vi "UniqueNameDialog.vi"(9 "Names in use":string[](array[string]), 10 "Device Name":string) -> (2 "Unique name":string)   [LabVIEW 2013]
doc: "Present dialog to ask for unique name, showing user list of reserved names."
uses:
  <vilib>/Utility/miscctls.llb/LVSelectionTypeDef.ctl
panel:
  out "unique?":bool
  in  "OK button":bool
  # "Please enter a unique name:"
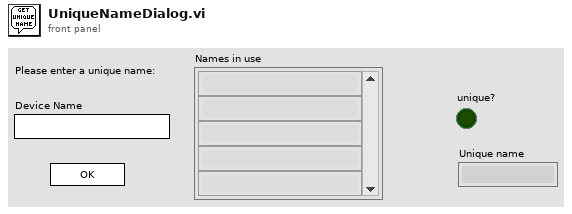
[diagram p1: front panel]
types:
  T1 = typedef "LVSelectionTypeDef.ctl" = cluster{"Selection Start":u32, "Selection End":u32}
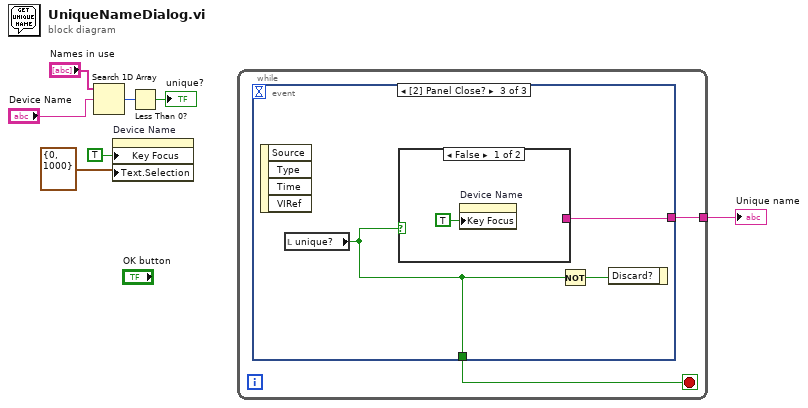
[diagram p0: block diagram]
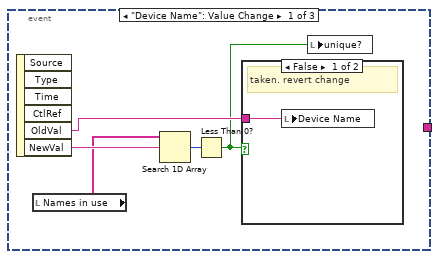
[diagram p2: hidden frame]
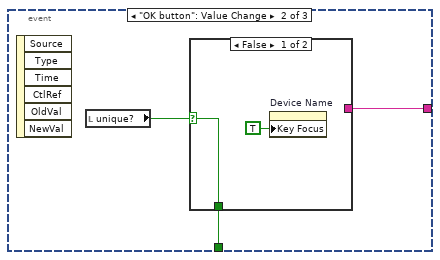
[diagram p4: hidden frame]
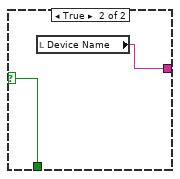
[diagram p5: hidden frame]
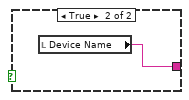
[diagram p6: hidden frame]
diagram:
  n1 = Search 1D Array(1D array="Names in use", element="Device Name") -> (index of element=w4:i32)  [unwired: 1 in]
  n2 = property on="Device Name" class="Str"("Key Focus"=TRUE, "Text.Selection"=T1 {"Selection Start"=0, "Selection End"=1000}) -> ()  [unwired: 2 in, 2 out]
  n3 = Less Than 0?(x=w4) -> (x < 0?=→"unique?":bool)
  n4 = while {
    tunnel: [w8] -> w7
    stop <- w9 stop-if-true
    n5 = event shown="[2] Panel Close?" {
      selector: _ -> [_ _ _]
      dyn-events: _ -> [_ _ _]
      timeout: _ -> [_ _ _]
      tunnel: [_ w16 w23] -> w9
      tunnel: [_ w17 w25] -> w8
      event "Device Name": Value Change {
        n6 = event-data() -> ("OldVal"=w11:string, "NewVal"=w14:string)  [unwired: 1 in, 4 out]
        n7 = local read "Names in use"() -> (w13:string[])
        n8 = Search 1D Array(1D array=w13, element=w14) -> (index of element=w12:i32)  [unwired: 1 in]
        n9 = Less Than 0?(x=w12) -> (x < 0?=w10:bool)
        n10 = case shown="False" w10 {
          tunnel: w11 -> [w15 _]
          frame False {
            # "taken. revert change"
            n11 = local write "Device Name"(w15) -> ()
          }
          frame True {
            # "unique!"
          }
        }
        n12 = local write "unique?"(w10) -> ()
      }
      event "OK button": Value Change {
        n13 = event-data() -> ()  [unwired: 1 in, 6 out]
        n14 = local read "unique?"() -> (w18:bool)
        n15 = case shown="False" w18 {
          selector: w18 -> [w19 w22]
          tunnel: [_ w21] -> w17
          tunnel: [w19 w22] -> w16
          frame False {
            n16 = property on="Device Name" class="Str"("Key Focus"=TRUE) -> ()  [unwired: 2 in, 2 out]
          }
          frame True {
            n17 = local read "Device Name"() -> (w21:string)
          }
        }
      }
      event Panel Close? {
        n18 = event-data() -> ()  [unwired: 1 in, 4 out]
        n19 = local read "unique?"() -> (w23:bool)
        n20 = case shown="False" w23 {
          tunnel: [_ w27] -> w25
          frame False {
            n21 = property on="Device Name" class="Str"("Key Focus"=TRUE) -> ()  [unwired: 2 in, 2 out]
          }
          frame True {
            n22 = local read "Device Name"() -> (w27:string)
          }
        }
        n23 = Not(x=w23) -> (.not. x?=w24:bool)
        n24 = event-data("Discard?"=w24) -> ()  [unwired: 1 in, 1 out]
      }
    }
  }
  "Unique name" <- w7
